vi "module_param.vi"() -> ()   [LabVIEW 2018]
panel:
  in  "module address":u8
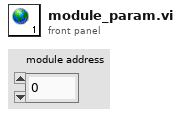
[diagram p1: front panel]
diagram:
